vi "SCD Get Infos.vi"(8 "error in (no error)":errorcluster) -> (0 "error out":errorcluster)   [LabVIEW 2020, in "Examples.lvlib"]
uses:
  Examples.lvlib
  Classes/SCD/SCD.lvclass
panel:
  out "firmwareVersion":string
  out "fpgaVersion":string
  out "boardRevision":string
  out "serialNumber":string
  # "Connector Pane"
  # "Locals"
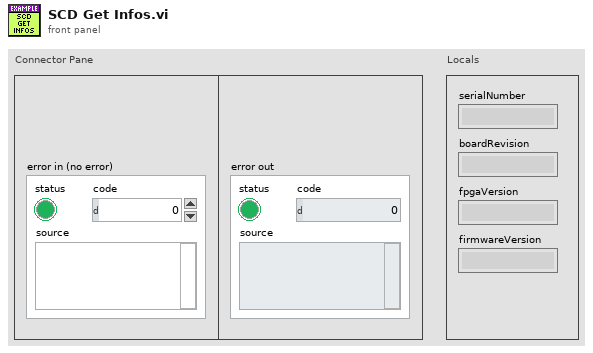
[diagram p1: front panel]
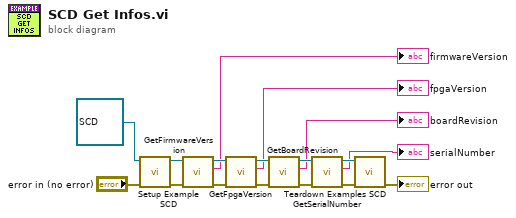
[diagram p0: block diagram]
diagram:
  n1 = call "Setup Example SCD.vi"("error in (no error)"="error in (no error)", "SCD in"=refnum<class "SCD.lvclass"> refnum) -> ("error out"=w15:errorcluster, "SCD out"=w16:refnum<class "SCD.lvclass">)  [unwired: 6 in, 2 out]
  n2 = call "GetFirmwareVersion.vi"("error in (no error)"=w15, "SCD in"=w16) -> ("error out"=w13:errorcluster, "firmwareVersion"=→"firmwareVersion":string, "SCD out"=w14:refnum<class "SCD.lvclass">)  [unwired: 7 in]
  n3 = call "GetFpgaVersion.vi"("error in (no error)"=w13, "SCD in"=w14) -> ("error out"=w11:errorcluster, "fpgaVersion"=→"fpgaVersion":string, "SCD out"=w12:refnum<class "SCD.lvclass">)  [unwired: 7 in]
  n4 = call "GetBoardRevision.vi"("error in (no error)"=w11, "SCD in"=w12) -> ("error out"=w9:errorcluster, "boardRevision"=→"boardRevision":string, "SCD out"=w10:refnum<class "SCD.lvclass">)  [unwired: 7 in]
  n5 = call "GetSerialNumber.vi"("error in (no error)"=w9, "SCD in"=w10) -> ("error out"=w7:errorcluster, "serialNumber"=→"serialNumber":string, "SCD out"=w8:refnum<class "SCD.lvclass">)  [unwired: 7 in]
  n6 = call "Teardown Examples SCD.vi"("error in (no error)"=w7, "Monochromator in"=w8) -> ("error out"=→"error out":errorcluster)  [unwired: 9 in]
